vi "Initialize Routing and Faulting Custom Device.vi"(8 "error in (no error)":errorcluster, 11 "RaF CD Ref in":T1 format="%.0x") -> (0 "error out":errorcluster, 1 "Aliases Section Ref":T1 format="%.0x", 2 "Routes Section Ref":T1 format="%.0x", 3 "RaF CD Ref out":T1 format="%.0x")   [LabVIEW 2017, in "Switch Scripting.lvlib"]
uses:
  Switch Scripting.lvlib
  <vilib>/NI Veristand/Custom Device API/Custom Device Item Ref.ctl
  Shared/Constants.vi
  <vilib>/NI VeriStand/Custom Device API/Custom Device API.lvlib
  Shared/Routing and Faulting Shared.lvlib
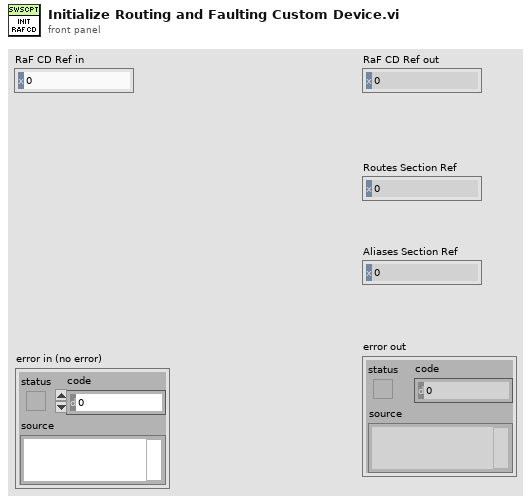
[diagram p1: front panel]
types:
  T1 = typedef "Custom Device API.lvlib/Custom Device Item Ref.ctl" = u64
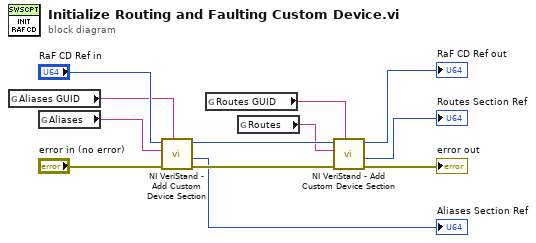
[diagram p0: block diagram]
diagram:
  n1 = global read "Constants.vi" "Aliases GUID"() -> (w2:string)
  n2 = global read "Constants.vi" "Aliases"() -> (w4:string)
  n3 = call <vilib>:"NI VeriStand - Add Custom Device Section.vi"("GUID (Default Section)"=w2, "error in (no error)"="error in (no error)", "Section Name"=w4, "Parent Ref in"="RaF CD Ref in") -> ("error out"=w11:errorcluster, "Section Ptr"=→"Aliases Section Ref":T1, "Parent Ref out"=w12:T1)  [unwired: 4 in, 1 out]
  n4 = global read "Constants.vi" "Routes GUID"() -> (w1:string)
  n5 = global read "Constants.vi" "Routes"() -> (w3:string)
  n6 = call <vilib>:"NI VeriStand - Add Custom Device Section.vi"("GUID (Default Section)"=w1, "error in (no error)"=w11, "Section Name"=w3, "Parent Ref in"=w12) -> ("error out"=→"error out":errorcluster, "Section Ptr"=→"Routes Section Ref":T1, "Parent Ref out"=→"RaF CD Ref out":T1)  [unwired: 4 in, 1 out]
